vi "fake lever.vi"() -> ()   [LabVIEW 2017]
uses:
  shake-parameters.ctl
  <vilib>/event_ctls.llb/eventvkey.ctl
  lorentzian.ctl
  circle corners.ctl
  four-corner circle transformation.ctl
  publisher action.ctl
  cursor action.ctl
  Q -- check range -- i -- real.vi
  Q - not nan -- real.vi
  cursor window action.ctl
  cursor winow.ctl
panel:
  in  "all":enum32{"all", "other"}(tab)
  in  "total exp time (sec)":dbl=2000.0 format="%#_10f"
  in  "total number of point":dbl=50000.0 format="%#_10f"
  out "dt (sec)":dbl=0.04 format="%#_10f"
  out "Plot: circle sweep window":cluster{dbl[], dbl[]}[](graph)
  out "dev out":cdb=0.007784300010942506-0.00030343700337688914i format="%#_10f"
  out "zi frreq":dbl=45226.18608374177 format="%#.2f"
  out "dev frreq":dbl=45097.91728454601 format="%#.3f"
  out "off freq":dbl=128.2687991957573 format="%#.2f"
  out "time(sec)":dbl=1321.7460808799951 format="%#_5f"
  in  "dev pars":T1={"base (Hz)"=45000.0, "period(sec)"=100.0, "amp (Hz)"=100.0, "G base (Hz)"=10.0, "G period(sec)"=4.0, "G amp (Hz)"=0.0, "B base (V)"=0.0, "B period(sec)"=40.0, " B amp (V)"=0.0} {"B amp (V)" format="%#_10f"; "B period(sec)" format="%#_10f"; "B base (V)" format="%#_10f"; "G amp (Hz)" format="%#_10f"; "G period(sec)" format="%#_10f"; "G base (Hz)" format="%#_10f"; "amp (Hz)" format="%#_10f"; "period(sec)" format="%#_10f"; "base (Hz)" format="%#_10f"}
  in  "lorentzian -- basic":T2={"Amplitude"=1.0, "omega(0)"=1000.0, "Gamma"=3.0, "phase"=0.0, "Q"=300.0, "Norm  Ampl"=nan, "z (inf)"=0.0+0.0i, "4corners"={"z (-pi/2)"=9.277908004825974e-07+0.0007240755403629966i, "z(inf)"=2.6527949823343002e-05+0.0007477540585896028i, "z (pi/2)"=2.8494315967368497e-06+0.0007733542176124632i, "z center"=1.8886111986097237e-06+0.0007487148789877299i, "z(0)"=-2.2750727426123552e-05+0.000749675699385857i, "radius"=2.4658065287076567e-05}} {"z (inf)" format="%#9_9f"; "Q" format="%#9_9f"; "phase" format="%#9_9f"; "Gamma" format="%#9_9f"; "omega(0)" format="%#9_9f"}
  out "Char":i16=50
  out "VKey":T4
  # "Gamma"
  # "backgr"
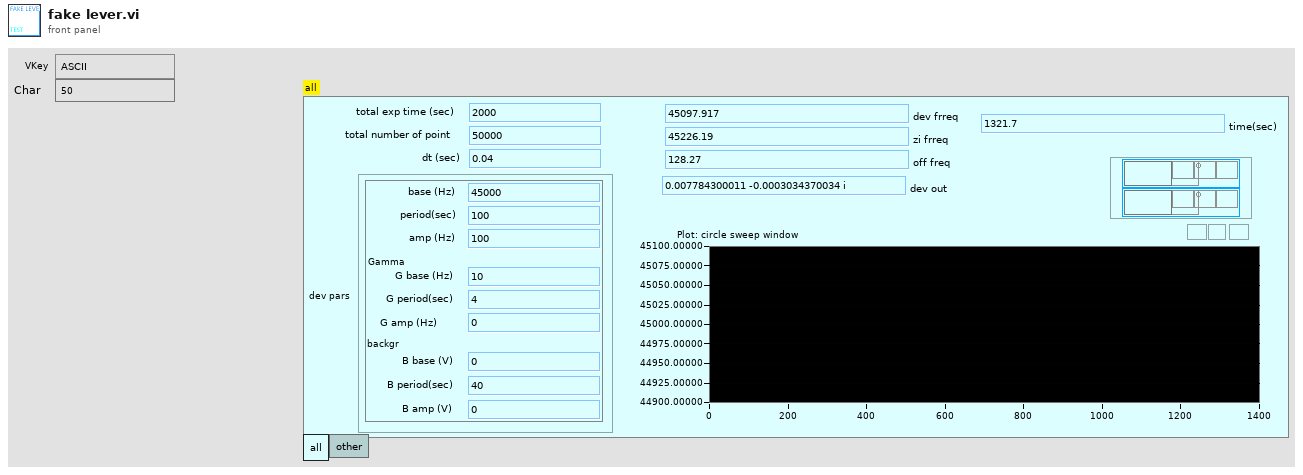
[diagram p1: front panel]
types:
  T1 = typedef "shake-parameters.ctl" = cluster{"base (Hz)":dbl, "period(sec)":dbl, "amp (Hz)":dbl, "G base (Hz)":dbl, "G period(sec)":dbl, "G amp (Hz)":dbl, "B base (V)":dbl, "B period(sec)":dbl, " B amp (V)":dbl}
  T2 = typedef "lorentzian.ctl" = cluster{"Amplitude":dbl, "omega(0)":dbl, "Gamma":dbl, "phase":dbl, "Q":dbl, "Norm  Ampl":dbl, "z (inf)":cdb, "4corners":T3}
  T3 = typedef "circle corners.ctl" = cluster{"z (-pi/2)":cdb, "z(inf)":cdb, "z (pi/2)":cdb, "z center":cdb, "z(0)":cdb, "radius":dbl}
  T4 = typedef "eventvkey.ctl" = enum16{"ASCII", "Enter", "Return", "Shift", "Ctrl", "Alt", "Cmd", "Opt", "Caps", "NumLock", "Clear", "Break", "Up", "Down", "Left", "Right", "Insert", "Delete", "Home", "End", "PageUp", "PageDown", "Escape", "Help", "Pause", "ScrollLock", "F1", "F2", "F3", "F4", "F5", "F6", "F7", "F8", "F9", "F10", "F11", "F12", "F13", "F14", "F15", "F16", "F17", "F18", "F19", "F20", "F21", "F22", "F23", "F24", "Play", "VolumeUp", "VolumeDown", "Mute", "Two Byte Char"}
  T5 = typedef "cursor winow.ctl" = cluster{"left":dbl, "right ":dbl, "center":dbl, "window":dbl, "cursors":i32[], "relative":i32, "absolute":i32, "fixed vertical offset":dbl, "vertical offset":dbl, "skew":dbl, "default window frac":dbl, "kind":enum16{"symmetric", "skewed", "fancy"}, "skew.left":dbl, "skew.right":dbl, "Plot ref":refnum<vi>, "wing order":enum16{"forw", "back"}}
  T6 = typedef "cursor window action.ctl" = enum16{"balance", "h. offset change", "cursor moves", "change center", "change window", "init", "check", "reset", "set y to middle", "idle", "-write all Y", "-write left.X", "-write center.X", "-write right.X", "-write all X", "-change center", "-change window", "-change skew", "-read cursor 2", "-read cursor 1", "-read cursor 0", "-read all cursors", "-reset", "-read plot scale", "-set y to middle", "-Q: center.Y is visible", "-Q: window is visible", "-parse center.Y", "-right left from center", "-left move", "-right move", "-set center.Y", "-empty", "-set cursors to default", "-check", "-write center.Y", "-copy cursor 1", "-copy cursor 0", "-copy cursor 2", "move right", "move left", "shrink", "broaden", "skew up", "skew down", "-write plot scale", "zoom X", "change cen&win", "zoom to all data", "color--red", "color--green", "color--yellow", "read", "zoom out", "zoom in", "slide right", "slide left", "set range aspect ratio to 1"}
  T7 = typedef "cursor action.ctl" = enum16{"range", "read", "write", "check", "zoom out", "smart zoom out", "zoom to aspect ratio 1", "zoom to win", "zoom out 20%", "zoom in 20%"}
  T8 = typedef "publisher action.ctl" = enum16{"set", "get"}
  T9 = typedef "four-corner circle transformation.ctl" = enum16{"z(c) z(inf)", "z(c) z(zero)", "fix phase", "calculate lorentzian", "z(0) z(+-pi/2)", "shift to zcenter", "to  canonical", "get canonical phase", "get4corners"}
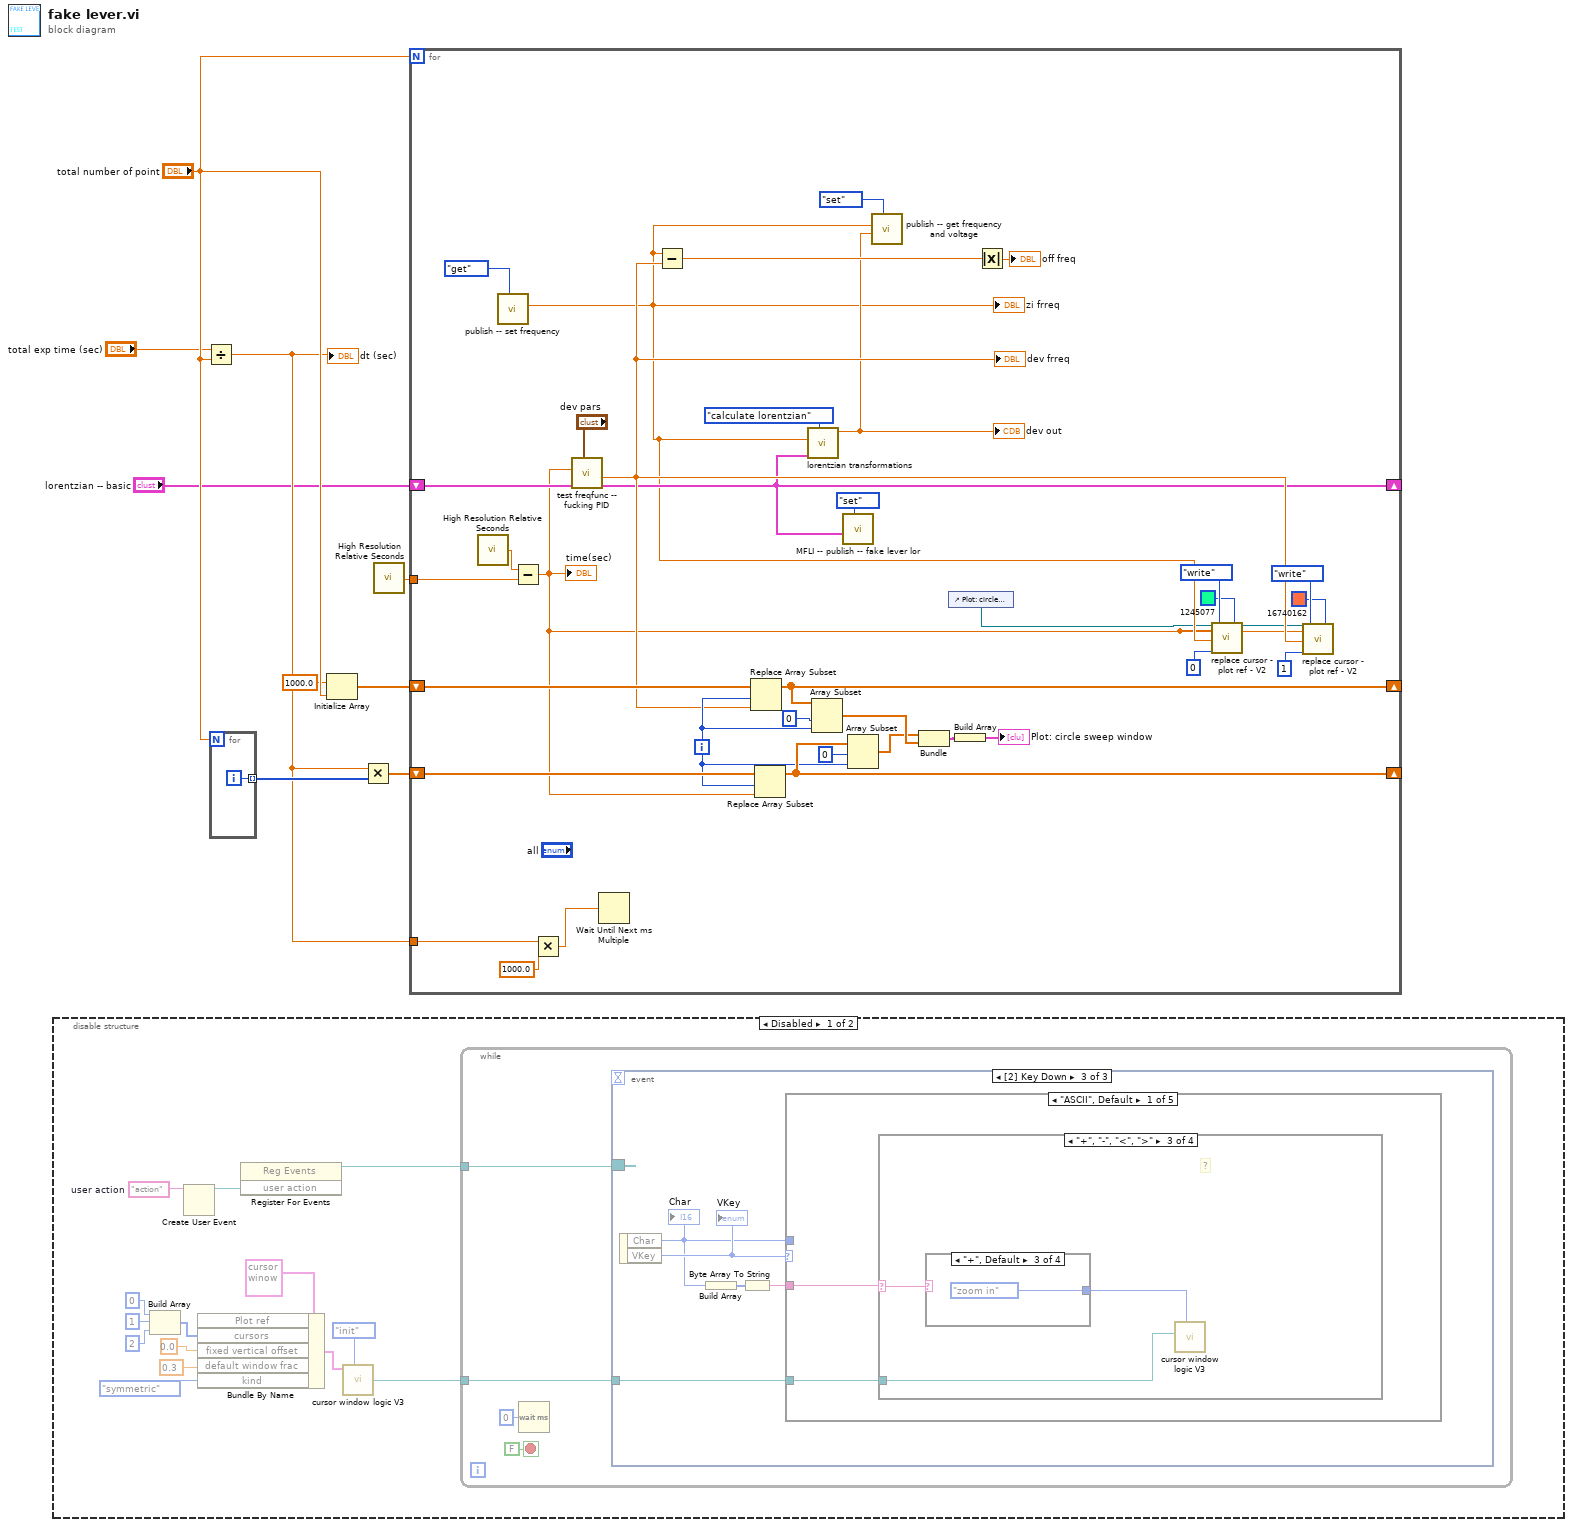
[diagram p0: block diagram]
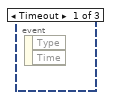
[diagram p2: hidden frame]
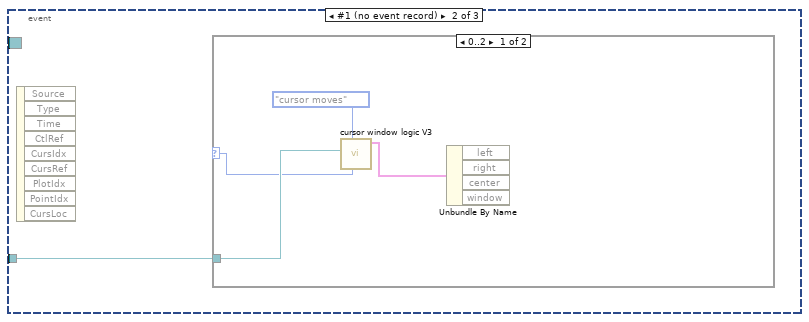
[diagram p3: hidden frame]
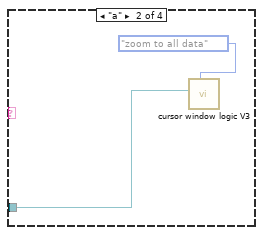
[diagram p6: hidden frame]
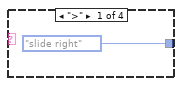
[diagram p7: hidden frame]
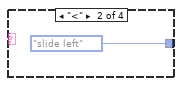
[diagram p8: hidden frame]
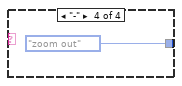
[diagram p9: hidden frame]
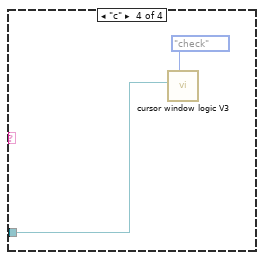
[diagram p10: hidden frame]
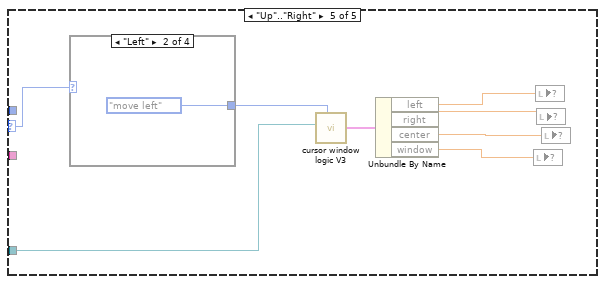
[diagram p14: hidden frame]
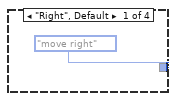
[diagram p15: hidden frame]
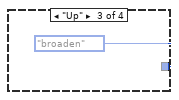
[diagram p16: hidden frame]
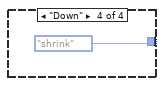
[diagram p17: hidden frame]
diagram:
  n1 = disable-structure shown="Disabled" {
    frame Disabled {
      w21 = "action"  # user action
      n2 = Build Array(0, 1, 2) -> (w10:i32[])
      n3 = Create User Event(user event datatype=w21) -> (user event=w22:refnum<user-event>)  [unwired: 1 in, 1 out]
      n4 = Bundle By Name(cluster=T5 {"left"=0.0, "right "=0.0, "center"=0.0, "window"=0.0, "cursors"=[], "relative"=0, "absolute"=0, "fixed vertical offset"=0.0, "vertical offset"=0.0, "skew"=0.0, "default window frac"=0.0, "kind"=enum."symmetric", "skew.left"=0.0, "skew.right"=0.0, "Plot ref"=refnum, "wing order"=enum."forw"} ("cursor bracket: All, data window"), "cursors"=w10, "fixed vertical offset"=0.0, "default window frac"=0.3 ("fixed vertical offset"), "kind"=enum16{"symmetric", "skewed", "fancy"}."symmetric") -> (w18:T5)  [unwired: 1 in]
      n5 = register-events(w22) -> (reference out=w20:refnum<event-registration>)  [unwired: 2 in, 1 out]
      n6 = call "cursor window logic V3.vi"("cursor window action"=cursor_window_action."init", "cursor window init"=w18) -> ("cursor window out"=w23:refnum<vi>)  [unwired: 8 in, 1 out]
      n7 = while {
        tunnel: w20 -> [w27]
        tunnel: w23 -> [w25]
        stop <- FALSE stop-if-true
        n8 = Wait (ms)(milliseconds to wait=u32 0) -> ()  [unwired: 1 out]
        n9 = event shown="[2] Key Down" {
          selector: w27 -> [_ _ _]
          dyn-events: _ -> [_ _ _]
          timeout: _ -> [_ _ _]
          tunnel: w25 -> [_ w28 w37]
          event Timeout {
            n10 = event-data() -> ()  [unwired: 1 in, 2 out]
          }
          event #1 (no event record) {
            n11 = event-data() -> ()  [unwired: 1 in, 9 out]
            n12 = case shown="0..2" {
              selector: _ -> [w34 _]
              tunnel: w28 -> [w36 _]
              frame 0..2 {
                n13 = call "cursor window logic V3.vi"("CursIdx"=w34, "cursor window action"=cursor_window_action."cursor moves", "cursor window in"=w36) -> ("cursor window out"=w33:T5)  [unwired: 7 in, 1 out]
                n14 = Unbundle By Name(w33) -> ("left"=w32:dbl, "right"=w31:dbl, "center"=w30:dbl, "window"=w29:dbl)
              }
              frame 3, Default {
              }
            }
          }
          event Key Down {
            n15 = event-data() -> ("Char"=w39:i16, "VKey"=w41:T4)  [unwired: 1 in]
            "Char" <- w39
            "VKey" <- w41
            n16 = Build Array(w39) -> (w40:i16[])
            n17 = Byte Array To String(unsigned byte array=w40) -> (string=w38:string)
            n18 = case shown="\"ASCII\", Default" w41 {
              selector: w41 -> [_ _ _ _ w62]
              tunnel: w39 -> [_ _ _ _ _]
              tunnel: w38 -> [w43 _ _ _ _]
              tunnel: w37 -> [w42 _ _ _ w55]
              frame "ASCII", Default {
                n19 = case shown="\"+\", \"-\", \"<\", \">\"" w43 {
                  selector: w43 -> [_ _ w47 _]
                  tunnel: w42 -> [_ w44 w48 w53]
                  frame "0", Default {
                  }
                  frame "a" {
                    n20 = call "cursor window logic V3.vi"("cursor window action"=cursor_window_action."zoom to all data", "cursor window in"=w44) -> ()  [unwired: 8 in, 2 out]
                  }
                  frame "+", "-", "<", ">" {
                    # "?"
                    n21 = case shown="\"+\", Default" w47 {
                      tunnel: [cursor_window_action."slide right" ("cursor window action") cursor_window_action."slide left" ("cursor window action") cursor_window_action."zoom in" ("cursor window action") cursor_window_action."zoom out" ("cursor window action")] -> w46
                      frame ">" {
                      }
                      frame "<" {
                      }
                      frame "+", Default {
                      }
                      frame "-" {
                      }
                    }
                    n22 = call "cursor window logic V3.vi"("cursor window action"=w46, "cursor window in"=w48) -> ()  [unwired: 8 in, 2 out]
                  }
                  frame "c" {
                    n23 = call "cursor window logic V3.vi"("cursor window action"=cursor_window_action."check", "cursor window in"=w53) -> ()  [unwired: 8 in, 2 out]
                  }
                }
              }
              frame "Escape" {
              }
              frame "PageUp" {
              }
              frame "PageDown" {
              }
              frame "Up".."Right" {
                n24 = case shown="\"Left\"" w62 {
                  tunnel: [cursor_window_action."move right" ("cursor window action") cursor_window_action."move left" ("cursor window action") cursor_window_action."broaden" ("cursor window action") cursor_window_action."shrink" ("cursor window action")] -> w57
                  frame "Right", Default {
                  }
                  frame "Left" {
                  }
                  frame "Up" {
                  }
                  frame "Down" {
                  }
                }
                n25 = call "cursor window logic V3.vi"("cursor window action"=w57, "cursor window in"=w55) -> ("cursor window out"=w56:T5)  [unwired: 8 in, 1 out]
                n26 = Unbundle By Name(w56) -> ("left"=w61:dbl, "right"=w60:dbl, "center"=w59:dbl, "window"=w58:dbl)
                n27 = local write item#-1(w58) -> ()
                n28 = local write item#-1(w61) -> ()
                n29 = local write item#-1(w60) -> ()
                n30 = local write item#-1(w59) -> ()
              }
            }
          }
        }
      }
    }
    frame Enabled {
    }
  }
  n31 = Divide(x="total exp time (sec)", y="total number of point") -> (x/y=w4:dbl)
  "dt (sec)" <- w4
  n32 = for {
    N: "total number of point" -> [_]
    tunnel: [w67] -> w6 mode=indexing
    i -> [w67]
  }
  n33 = Initialize Array(1000.0 ("element"), "total number of point") -> (w2:dbl[])
  n34 = Multiply(x=w4, y=w6) -> (x*y=w5:dbl[])
  n35 = call <vilib>:"High Resolution Relative Seconds.vi"() -> ("relative seconds"=w9:dbl)
  n36 = for {
    N: "total number of point" -> [_]
    shift-right: [w77] -> _
    shift-left: "lorentzian -- basic" -> [w86]
    tunnel: w9 -> [w104]
    shift-right: [w93] -> _
    shift-left: w2 -> [w103]
    shift-right: [w89] -> _
    shift-left: w5 -> [w102]
    tunnel: w4 -> [w100]
    i -> [w87]
    n37 = call <vilib>:"High Resolution Relative Seconds.vi"() -> ("relative seconds"=w101:dbl)
    n38 = call "publish -- set frequency.vi"("publisher action"=publisher_action."get") -> ("freq out (Hz)"=w73:dbl)  [unwired: 10 in]
    "zi frreq" <- w73
    n39 = Subtract(x=w101, y=w104) -> (x-y=w69:dbl)
    "time(sec)" <- w69
    n40 = Multiply(x=w100, y=1000.0) -> (x*y=w68:dbl)
    n41 = call "test freqfunc -- fucking PID.vi"("pars"="dev pars", "lorentzian -- basic"=w86, "time (sec)"=w69) -> ("lorentzian -- basic -- OUT"=w77:T2, "freq (Hz)"=w79:dbl)  [unwired: 7 in]
    "dev frreq" <- w79
    n42 = Wait Until Next ms Multiple(millisecond multiple=w68) -> ()  [unwired: 1 out]
    n43 = Subtract(x=w73, y=w79) -> (x-y=w83:dbl)
    n44 = Replace Array Subset(array=w103, new element=w79, index=w87) -> (w93:dbl[])
    n45 = Replace Array Subset(array=w102, new element=w69, index=w87) -> (w89:dbl[])
    n46 = call "lorentzian transformations.vi"("4 corner circle transformation"=four-corner_circle_transformation."calculate lorentzian", "lorentzian in"=w77, "freq in"=w73) -> ("voltage out"=w78:cdb)  [unwired: 6 in, 2 out]
    "dev out" <- w78
    n47 = Array Subset(array=w93, index=0 ("cursor index"), length=w87) -> (w91:dbl[])
    n48 = call "MFLI -- publish -- fake lever lor.vi"("publisher action"=publisher_action."set", "lorentzian IN"=w77) -> ()  [unwired: 9 in, 1 out]
    n49 = Array Subset(array=w89, index=0 ("cursor index"), length=w87) -> (w90:dbl[])
    n50 = call "publish -- get frequency and voltage.vi"("publisher action"=publisher_action."set", "Voltage IN (V)"=w78, "freq IN (Hz)"=w73) -> ()  [unwired: 7 in, 2 out]
    n51 = Bundle(w90, w91) -> (w97:cluster{dbl[], dbl[]})  [unwired: 1 in]
    n52 = control-ref of="Plot: circle sweep window"() -> (w71:refnum<vi>)
    n53 = Build Array(w97) -> (→"Plot: circle sweep window":cluster{dbl[], dbl[]}[])
    n54 = Absolute Value(x=w83) -> (abs(x)=→"off freq":dbl)
    n55 = call "replace cursor - plot ref - V2.vi"("Plot ref in"=w71, "new X"=w69, "new  Y"=w73, "cursor index"=0, "cursor action"=cursor_action."write", "Color Box"=u32 1245077) -> ("Plot ref out"=w70:refnum<vi>)  [unwired: 11 in, 2 out]
    n56 = call "replace cursor - plot ref - V2.vi"("Plot ref in"=w70, "new X"=w69, "new  Y"=w79, "cursor index"=1, "cursor action"=cursor_action."write", "Color Box"=u32 16740162) -> ()  [unwired: 11 in, 3 out]
  }
